vi "LOADread.vi"(8 "error in (no error)":errorcluster, 11 "VISA resource name":refnum<visa-resource-name>) -> (0 "error out":errorcluster, 1 "X":dbl, 2 "R":dbl, 3 "VISA resource name out":refnum<visa-resource-name>)   [LabVIEW 2016]
panel:
  in  "Enable Short Correction (F: Disable)":bool
  in  "Short Supplementary Threshold (0)":dbl
  in  "Short Capacitance Threshold (0)":dbl
  in  "Short Correction Type (0: Resistance- Reactance)":u16(ring) items=[" Resistance- Reactance", "Series Inductance- Series Resistance"]
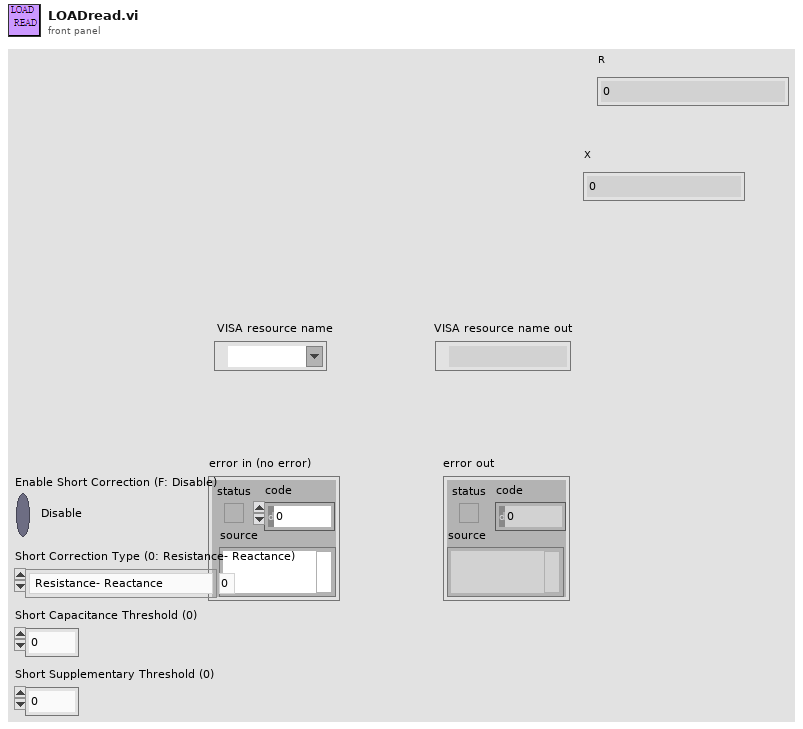
[diagram p1: front panel]
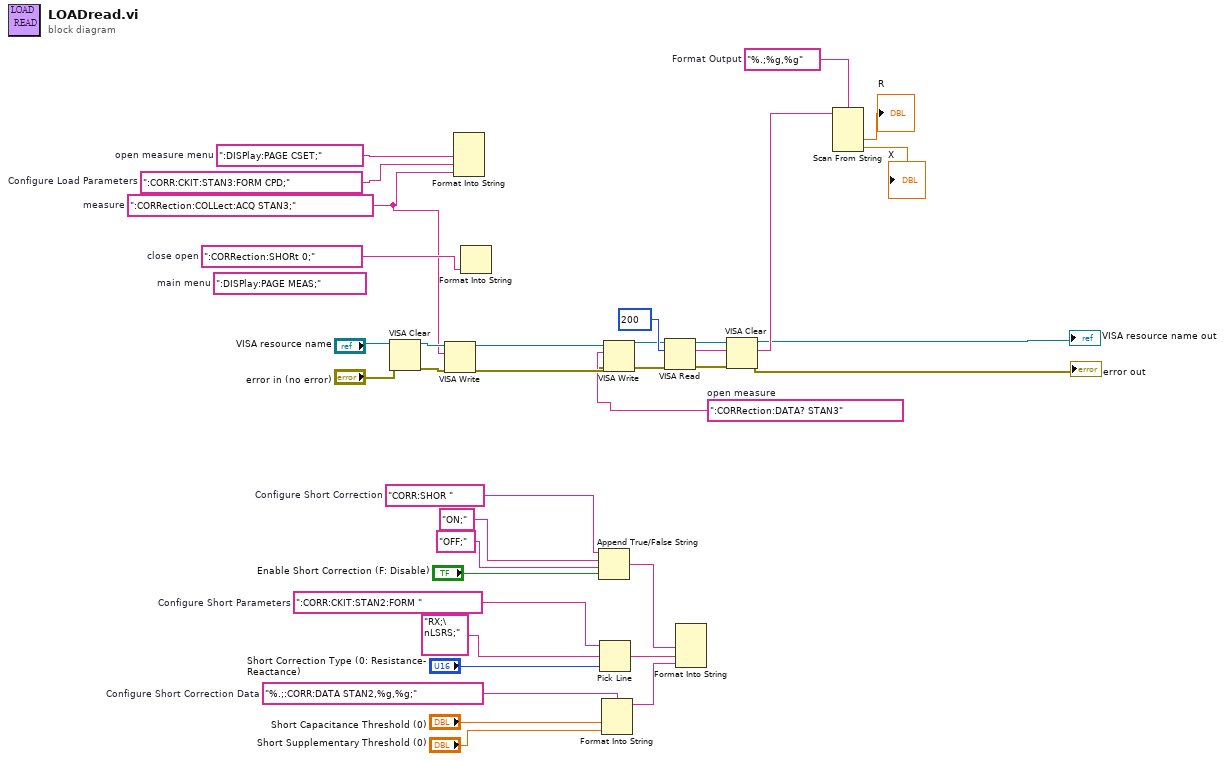
[diagram p0: block diagram]
diagram:
  w2 = ":CORR:CKIT:STAN3:FORM CPD;"  # Configure Load Parameters
  w8 = "%.;%g,%g"  # Format Output
  w14 = ":CORRection:DATA? STAN3"  # open measure
  w21 = ":CORRection:SHORt 0;"  # close open
  w1 = ":CORRection:COLLect:ACQ STAN3;"  # measure
  (unwired) ":DISPlay:PAGE MEAS;"  # main menu
  w22 = ":DISPlay:PAGE CSET;"  # open measure menu
  w27 = "%.;:CORR:DATA STAN2,%g,%g;"  # Configure Short Correction Data
  w31 = ":CORR:CKIT:STAN2:FORM "  # Configure Short Parameters
  w35 = "CORR:SHOR "  # Configure Short Correction
  n1 = VISA Clear(VISA resource name="VISA resource name", error in (no error)="error in (no error)") -> (VISA resource name out=w20:refnum<visa-resource-name>, error out=w19:errorcluster)
  n2 = VISA Write(VISA resource name=w20, write buffer=w1, error in (no error)=w19) -> (VISA resource name out=w16:refnum<visa-resource-name>, error out=w15:errorcluster)  [unwired: 1 out]
  n3 = Format Into String(w22, w2, w1) -> ()  [unwired: 3 in, 2 out]
  n4 = Format Into String(w21) -> ()  [unwired: 3 in, 2 out]
  n5 = Append True/False String(1:"Enable Short Correction (F: Disable)", 2:"OFF;" ("true string"), 3:"ON;" ("true string"), 4:w35) -> (0:w24:string)
  n6 = Pick Line(string ("")=w31, multi-line string="RX;\nLSRS;", line index="Short Correction Type (0: Resistance- Reactance)") -> (output string=w25:string)
  n7 = Format Into String(format string=w27, "Short Capacitance Threshold (0)", "Short Supplementary Threshold (0)") -> (resulting string=w23:string)  [unwired: 2 in, 1 out]
  n8 = VISA Write(VISA resource name=w16, write buffer=w14, error in (no error)=w15) -> (VISA resource name out=w11:refnum<visa-resource-name>, error out=w12:errorcluster)  [unwired: 1 out]
  n9 = VISA Read(VISA resource name=w11, byte count=u32 200, error in (no error)=w12) -> (VISA resource name out=w6:refnum<visa-resource-name>, read buffer=w7:string, error out=w5:errorcluster)  [unwired: 1 out]
  n10 = Format Into String(w24, w25, w23) -> ()  [unwired: 3 in, 2 out]
  n11 = VISA Clear(VISA resource name=w6, error in (no error)=w5) -> (VISA resource name out=→"VISA resource name out":refnum<visa-resource-name>, error out=→"error out":errorcluster)
  n12 = Scan From String(format string=w8, input string=w7) -> (output 1=→"R":dbl, output 2=→"X":dbl)  [unwired: 4 in, 3 out]
